vi "mro_getVersion.vi"(8 "error in (no error)":errorcluster, 11 "status in":i32) -> (0 "error out":errorcluster, 2 "version":string, 3 "status out":i32)   [LabVIEW 2011]
uses:
  mirao52e.dll
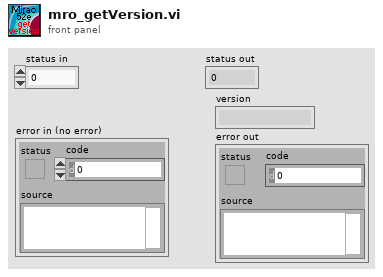
[diagram p1: front panel]
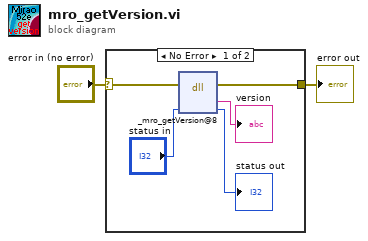
[diagram p0: block diagram]
diagram:
  n1 = case shown="No Error" "error in (no error)" {
    selector: "error in (no error)" -> [w5 w8]
    tunnel: [w4 w8] -> w1
    frame No Error {
      n2 = dll-call lib="C:/Users/myerslab/Documents/Tests/MiraoWrappers/mirao52e.dll" fn="_mro_getVersion@8"(error in=w5, "status"="status in") -> (error out=w4:errorcluster, "version"=→"version":string, "status"=→"status out":i32)  [unwired: 4 in, 1 out]
    }
    frame Error {
    }
  }
  "error out" <- w1
